vi "Parse Datagram.vi"(4 "source address":u32, 6 "source port":u16, 7 "transfer group id":i32, 8 "error in (no error)":errorcluster, 10 "datagram":string, 11 "UDPlog Transceiver in":refnum<class "UDPlog Transceiver.lvclass">) -> (0 "error out":errorcluster, 1 "valid":bool, 2 "transfer data":string, 3 "UDPlog Transceiver out":refnum<class "UDPlog Transceiver.lvclass">, 5 "transfer id":i32)   [LabVIEW 2023, in "UDPlog.lvlib" / "UDPlog Transceiver.lvclass"]
uses:
  UDPlog Transceiver.lvclass
  UDPlog Transceiver.lvclass/UDPlog Transceiver.ctl
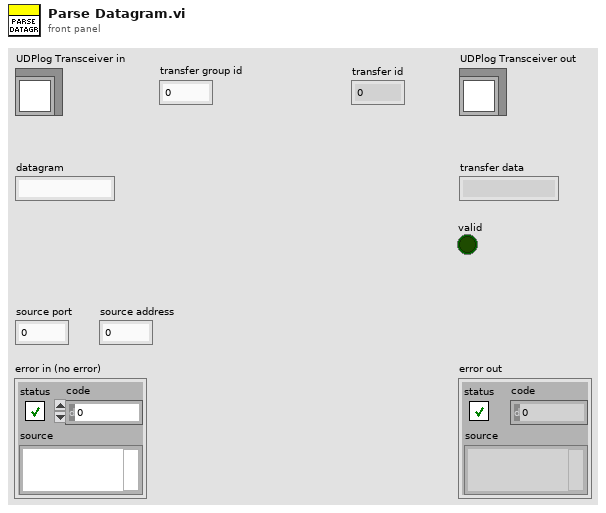
[diagram p1: front panel]
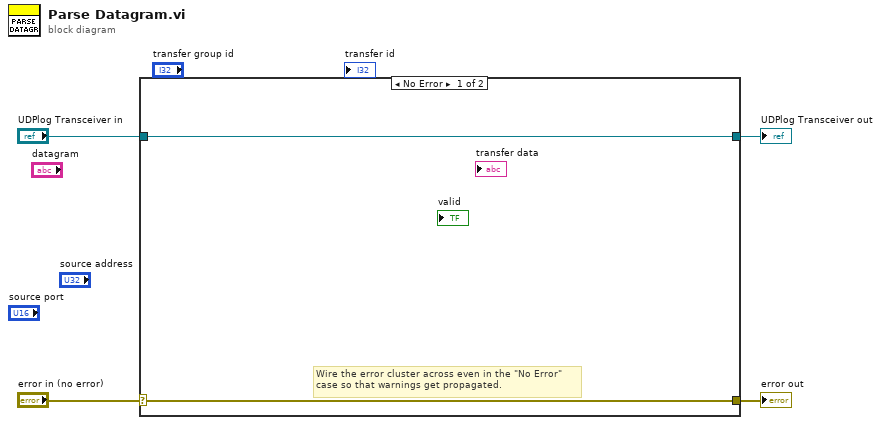
[diagram p0: block diagram]
diagram:
  n1 = case shown="No Error" "error in (no error)" {
    selector: "error in (no error)" -> [w5 w8]
    tunnel: [w5 w8] -> w3
    tunnel: [w6 w7] -> w1
    tunnel: "UDPlog Transceiver in" -> [w6 w7]
    frame No Error {
      # "Wire the error cluster across even in the \"No Error\"\ncase so that warnings get propagated."
    }
    frame Error {
    }
  }
  "error out" <- w3
  "UDPlog Transceiver out" <- w1
